vi "Numeric Functions Perfect Number.vi"() -> ()   [LabVIEW 2019]
panel:
  out "Perfect Number":dbl
  in  "Prime Number n":dbl
  # "Challenge:\nPerfect numbers. Write a program that accepts a prime number n and uses it to calculate a perfect number that has the form (2^n - 1) (2^(n-1)). Note: You can use the Mersenne Prime challenge program as a start."
  # "Try it: Enter a prime number in the \"Prime Number n\" box and hit Run."
  # "You will probably need:\nControls, indicators, and constants. numeric functions."
  # "Open the block diagram to see a possible solution."
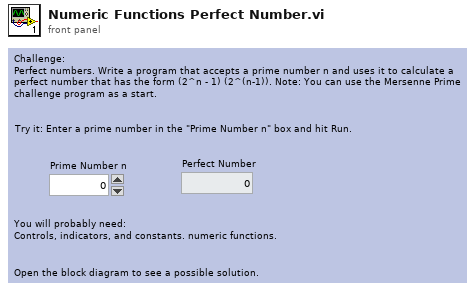
[diagram p1: front panel]
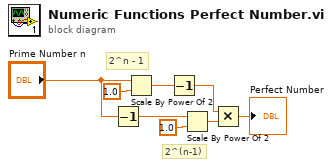
[diagram p0: block diagram]
diagram:
  # "2^(n-1)"
  # "2^n - 1"
  n1 = Decrement(x="Prime Number n") -> (x-1=w4:dbl)
  n2 = Scale By Power Of 2(n="Prime Number n", x=1.0) -> (x*2^n=w7:dbl)
  n3 = Decrement(x=w7) -> (x-1=w3:dbl)
  n4 = Scale By Power Of 2(n=w4, x=1.0) -> (x*2^n=w2:dbl)
  n5 = Multiply(x=w3, y=w2) -> (x*y=→"Perfect Number":dbl)
